vi "GetTemplate.vi"(11 "ListBox in":refnum<vi>) -> (4 "Python":string)   [LabVIEW 2016]
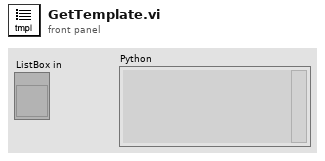
[diagram p1: front panel]
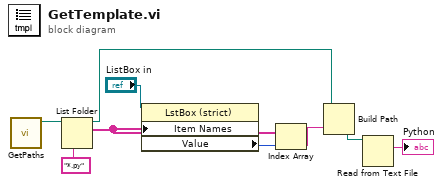
[diagram p0: block diagram]
diagram:
  n1 = call "GetPaths.vi"() -> ("Templates path"=w2:path)  [unwired: 10 in, 1 out]
  n2 = List Folder(path=w2, pattern="*.py") -> (path out=w5:path, filenames=w7:string[])  [unwired: 2 in, 2 out]
  n3 = property on="Property Node" class="LstBox (strict)"(reference="ListBox in", "Item Names"=w7) -> ("Value"=w1:i32)  [unwired: 1 in, 2 out]
  n4 = Index Array(array=w7, index=w1) -> (element=w6:string)
  n5 = Build Path(base path=w5, name or relative path=w6) -> (appended path=w3:path)
  n6 = Read from Text File(file (use dialog)=w3) -> (text=→"Python":string)  [unwired: 3 in, 3 out]
